vi "Voorbeeld_State_Machine.vi"() -> ()   [LabVIEW 2019]
panel:
  in  "State 1 of State 2":bool
  in  "stop":bool
  out "String":string
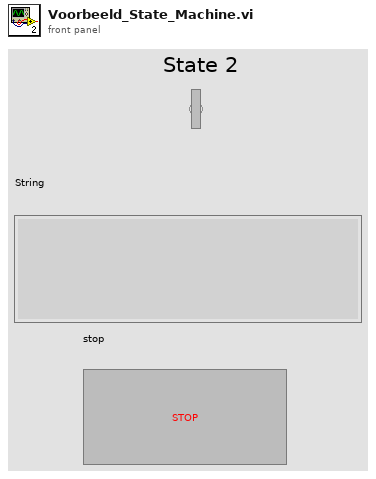
[diagram p1: front panel]
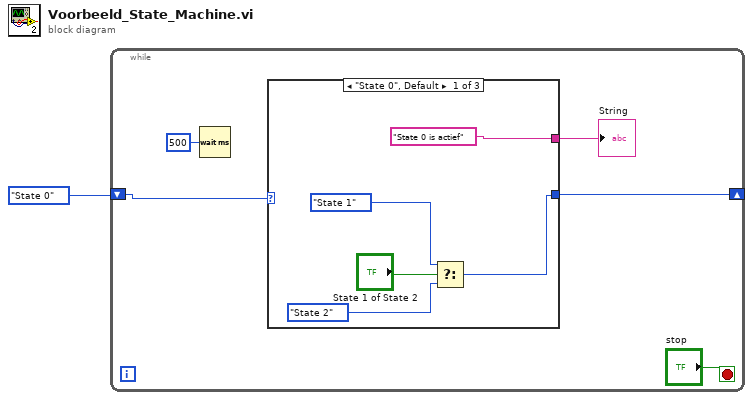
[diagram p0: block diagram]
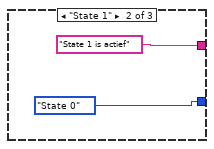
[diagram p2: hidden frame]
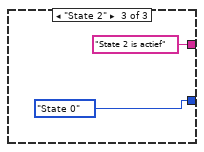
[diagram p3: hidden frame]
diagram:
  n1 = while {
    shift-right: [w3] -> _
    shift-left: enum16{"State 0", "State 1", "State 2"}."State 0" -> [w5]
    stop <- "stop" stop-if-true
    n2 = Wait (ms)(milliseconds to wait=u32 500) -> ()  [unwired: 1 out]
    n3 = case shown="\"State 0\", Default" w5 {
      tunnel: ["State 0 is actief" ("String") "State 1 is actief" ("String") "State 2 is actief" ("String")] -> w4
      tunnel: [w8 enum16{"State 0", "State 1", "State 2"}."State 0" enum16{"State 0", "State 1", "State 2"}."State 0"] -> w3
      frame "State 0", Default {
        n4 = Select(t=enum16{"State 0", "State 1", "State 2"}."State 1", s="State 1 of State 2", f=enum16{"State 0", "State 1", "State 2"}."State 2") -> (s? t:f=w8:enum16{"State 0", "State 1", "State 2"})
      }
      frame "State 1" {
      }
      frame "State 2" {
      }
    }
    "String" <- w4
  }
